vi "VI Main 1.1GPIB.vi"() -> ()   [LabVIEW 2014]
uses:
  <vilib>/Utility/file.llb/Write To Spreadsheet File (DBL).vi
  <vilib>/Analysis/NI_AALPro.lvlib
panel:
  in  "Save to File":bool
  in  "file path (dialog if empty)":path
  in  "clear graph at start":bool=TRUE
  in  "clear graph":bool
  out "Elapsed Time":dbl=5.100291728973389 format="%<%H:%M:%S>t"
  out "Measuring!":bool
  out "Current Interval":i32=2
  out "Benchmark (s)":dbl=1.077 format="%.2g"
  out "Start time":timestamp=timestamp(3634319869.0891385 s since 1904-01-01)
  in  "STOP acq":bool
  in  "# of Intervals":i32=20 min=2 step=1
  in  "Interval (s)":dbl=3.0 min=1.0 step=1.0
  in  "Quick Acq":bool
  in  "Multi Acq":bool
  in  "Reset":bool
  in  "Single Acq":bool
  in  "stop":bool
  out "intercept":dbl=5.632151768673284e-07 format="%_4g"
  out "Waveform Chart":dbl(graph)=1498.8953969009954
  out "Res. (ohm)":dbl=1498.8953969009954 format="%#.5g"
  out "XY Graph":cluster{dbl[], "Best Linear Fit":dbl[]}[](graph)=[{[0.0, 0.05050000175833702, 0.10100000351667404, 0.15150000154972076, 0.20200000703334808, 0.2524999976158142, 0.30300000309944153, 0.35350000858306885, 0.40400001406669617, 0.4544999897480011, 0.5049999952316284, 0.5554999709129333, 0.6060000061988831, 0.656499981880188, 0.7070000171661377, 0.7574999928474426, 0.8080000281333923, 0.8585000038146973, 0.9089999794960022, 0.9595000147819519, 1.0099999904632568, 1.0605000257492065, 1.1109999418258667, 1.1614999771118164, 1.2120000123977661, 1.2625000476837158, 1.312999963760376, 1.3634999990463257, 1.4140000343322754, 1.4644999504089355, 1.5149999856948853, 1.565500020980835, 1.6160000562667847, 1.6664999723434448, 1.7170000076293945, 1.7675000429153442, 1.8179999589920044, 1.868499994277954, 1.9190000295639038, 1.969499945640564, 2.0199999809265137, 2.070499897003174, 2.121000051498413, 2.1714999675750732, 2.2219998836517334, 2.2725000381469727, 2.322999954223633, 2.373500108718872, 2.4240000247955322, 2.4744999408721924, 2.5255000591278076, 2.5759999752044678, 2.626499891281128, 2.677000045776367, 2.7274999618530273, 2.7780001163482666, 2.8285000324249268, 2.878999948501587, 2.929500102996826, 2.9800000190734863, 3.0304999351501465, 3.0810000896453857, 3.131500005722046, 3.181999921798706, 3.2325000762939453, 3.2829999923706055, 3.3334999084472656, 3.384000062942505, 3.434499979019165, 3.484999895095825, 3.5355000495910645, 3.5859999656677246, 3.6364998817443848, 3.687000036239624, 3.737499952316284, 3.7880001068115234, 3.8385000228881836, 3.8889999389648438, 3.939500093460083, 3.990000009536743, 4.040500164031982, 4.091000080108643, 4.141499996185303, 4.191999912261963, 4.242499828338623, 4.293000221252441, 4.343500137329102, 4.394000053405762, 4.444499969482422, 4.494999885559082, 4.545499801635742, 4.5960001945495605, 4.646500110626221, 4.697000026702881, 4.747499942779541, 4.797999858856201, 4.848499774932861, 4.89900016784668, 4.94950008392334, 5.0], "Best Linear Fit"=[2.9321361694201187e-07, 3.4316144592594355e-05, 6.788442260585725e-05, 0.00010163152910536155, 0.0001353666593786329, 0.0001692490477580577, 0.00020289691747166216, 0.0002365230757277459, 0.0002702110796235502, 0.0003039317671209574, 0.0003375497763045132, 0.00037135041202418506, 0.00040501810144633055, 0.000438651826698333, 0.0004723611054942012, 0.0005059913382865489, 0.0005397166823968291, 0.0005734616424888372, 0.0006071235402487218, 0.0006408520275726914, 0.000674474285915494, 0.0007079437491483986, 0.0007418016903102398, 0.0007753406534902751, 0.0008092316566035151, 0.0008428616565652192, 0.0008766247192397714, 0.0009101884788833559, 0.0009441068395972252, 0.000977773917838931, 0.0010113242315128446, 0.00104525254573673, 0.0010786742204800248, 0.0011119291884824634, 0.0011458882363513112, 0.0011792887235060334, 0.0012128128437325358, 0.001246674102731049, 0.0012809749459847808, 0.0013138956855982542, 0.0013484194641932845, 0.0013821402098983526, 0.001415521022863686, 0.0014488088199868798, 0.0014823464443907142, 0.0015171199338510633, 0.0015507071511819959, 0.0015843959990888834, 0.0016174258198589087, 0.001652282546274364, 0.001685628667473793, 0.001718429964967072, 0.0017526380252093077, 0.0017857326893135905, 0.0018194534350186586, 0.001854273141361773, 0.0018880483694374561, 0.0019207267323508859, 0.0019549881108105183, 0.001989204902201891, 0.0020224947948008776, 0.002056337194517255, 0.0020900650415569544, 0.0021233297884464264, 0.0021574627608060837, 0.0021917179692536592, 0.0022237151861190796, 0.002258580643683672, 0.0022912463173270226, 0.0023252873215824366, 0.0023596647661179304, 0.0023923530243337154, 0.0024269770365208387, 0.0024603772908449173, 0.002494191052392125, 0.0025280059780925512, 0.0025607654824852943, 0.0025952423457056284, 0.0026286595966666937, 0.0026625576429069042, 0.002696041017770767, 0.002730145351961255, 0.0027635691221803427, 0.0027978394646197557, 0.00283193145878613, 0.0028640953823924065, 0.002898684237152338, 0.0029313690029084682, 0.002965638181194663, 0.0029995907098054886, 0.0030326275154948235, 0.0030669174157083035, 0.003100987756624818, 0.003135110717266798, 0.0031680287793278694, 0.0032008818816393614, 0.0032355813309550285, 0.003269442357122898, 0.0033022440038621426, 0.0033363213296979666]}, {[0.0, 0.05050000175833702, 0.10100000351667404, 0.15150000154972076, 0.20200000703334808, 0.2524999976158142, 0.30300000309944153, 0.35350000858306885, 0.40400001406669617, 0.4544999897480011, 0.5049999952316284, 0.5554999709129333, 0.6060000061988831, 0.656499981880188, 0.7070000171661377, 0.7574999928474426, 0.8080000281333923, 0.8585000038146973, 0.9089999794960022, 0.9595000147819519, 1.0099999904632568, 1.0605000257492065, 1.1109999418258667, 1.1614999771118164, 1.2120000123977661, 1.2625000476837158, 1.312999963760376, 1.3634999990463257, 1.4140000343322754, 1.4644999504089355, 1.5149999856948853, 1.565500020980835, 1.6160000562667847, 1.6664999723434448, 1.7170000076293945, 1.7675000429153442, 1.8179999589920044, 1.868499994277954, 1.9190000295639038, 1.969499945640564, 2.0199999809265137, 2.070499897003174, 2.121000051498413, 2.1714999675750732, 2.2219998836517334, 2.2725000381469727, 2.322999954223633, 2.373500108718872, 2.4240000247955322, 2.4744999408721924, 2.5255000591278076, 2.5759999752044678, 2.626499891281128, 2.677000045776367, 2.7274999618530273, 2.7780001163482666, 2.8285000324249268, 2.878999948501587, 2.929500102996826, 2.9800000190734863, 3.0304999351501465, 3.0810000896453857, 3.131500005722046, 3.181999921798706, 3.2325000762939453, 3.2829999923706055, 3.3334999084472656, 3.384000062942505, 3.434499979019165, 3.484999895095825, 3.5355000495910645, 3.5859999656677246, 3.6364998817443848, 3.687000036239624, 3.737499952316284, 3.7880001068115234, 3.8385000228881836, 3.8889999389648438, 3.939500093460083, 3.990000009536743, 4.040500164031982, 4.091000080108643, 4.141499996185303, 4.191999912261963, 4.242499828338623, 4.293000221252441, 4.343500137329102, 4.394000053405762, 4.444499969482422, 4.494999885559082, 4.545499801635742, 4.5960001945495605, 4.646500110626221, 4.697000026702881, 4.747499942779541, 4.797999858856201, 4.848499774932861, 4.89900016784668, 4.94950008392334, 5.0], "Best Linear Fit"=[5.632151768673284e-07, 3.425469348999516e-05, 6.794617180312299e-05, 0.00010163764763089373, 0.00013532912842937865, 0.0001690205992864352, 0.00020271208008492013, 0.00023640356088340506, 0.00027009504168188996, 0.0003037865025975182, 0.0003374779833960031, 0.00037116944431163135, 0.0004048609449929729, 0.00043855240590860115, 0.0004722439065899428, 0.000505935367505571, 0.0005396268681869126, 0.0005733183291025409, 0.0006070097900181691, 0.0006407012906995107, 0.0006743927516151388, 0.0007080842522964805, 0.0007417756734463953, 0.0007754671741277369, 0.0008091586748090786, 0.0008428501754904202, 0.000876541596640335, 0.0009102330973216766, 0.0009439245980030183, 0.000977616019152933, 0.0010113075198342747, 0.0010449990205156163, 0.001078690521196958, 0.0011123819423468728, 0.0011460734430282144, 0.001179764943709556, 0.0012134563648594707, 0.0012471478655408123, 0.001280839366222154, 0.0013145307873720688, 0.0013482222880534104, 0.0013819137092033252, 0.0014156052894160936, 0.0014492967105660085, 0.0014829881317159233, 0.0015166797119286917, 0.0015503711330786066, 0.001584062713291375, 0.0016177541344412898, 0.0016514455555912046, 0.0016854706906080038, 0.0017191621117579187, 0.0017528535329078335, 0.001786545113120602, 0.0018202365342705167, 0.0018539281144832852, 0.0018876195356332, 0.0019213109567831148, 0.001955002536995883, 0.001988693958145798, 0.0020223853792957127, 0.0020560769595084813, 0.002089768380658396, 0.002123459801808311, 0.002157151382021079, 0.0021908428031709943, 0.002224534224320909, 0.0022582258045336775, 0.002291917225683592, 0.002325608646833507, 0.0023593002270462754, 0.00239299164819619, 0.002426683069346105, 0.0024603746495588733, 0.0024940660707087883, 0.0025277576509215565, 0.0025614490720714716, 0.002595140493221386, 0.002628832073434155, 0.0026625234945840694, 0.002696215074796838, 0.0027299064959467527, 0.0027635979170966677, 0.0027972893382465823, 0.0028309807593964974, 0.002864672498672119, 0.0028983639198220342, 0.002932055340971949, 0.002965746762121864, 0.0029994381832717785, 0.0030331296044216935, 0.0030668213436973154, 0.0031005127648472304, 0.003134204185997145, 0.0031678956071470596, 0.0032015870282969747, 0.0032352784494468893, 0.0032689701887225115, 0.003302661609872426, 0.003336353031022341]}]
  in  "Sense range":i32(slide)
  in  "Stop (V)":dbl=5.0 format="%.4f"
  in  "Source compliance (A)":dbl=0.01 format="%.4f"
  in  "Direction":i32(slide)
  in  "Ranging":i32(slide)
  in  "Start (V)":dbl step=1.0 format="%.4p"
  in  "# of points to acquire":i32=50 min=1 max=2500 step=1
  in  "Speed":i32(slide)=2
  out "status":i32 format="%.0x"
  in  "resource name 2":string="GPIB0::24::INSTR"
  out "Qrun":bool
  out "Mrun":bool
  out "Srun":bool
  # ">"
  # "by L.Andrzejewski\nlandrzej@uottawa.ca"
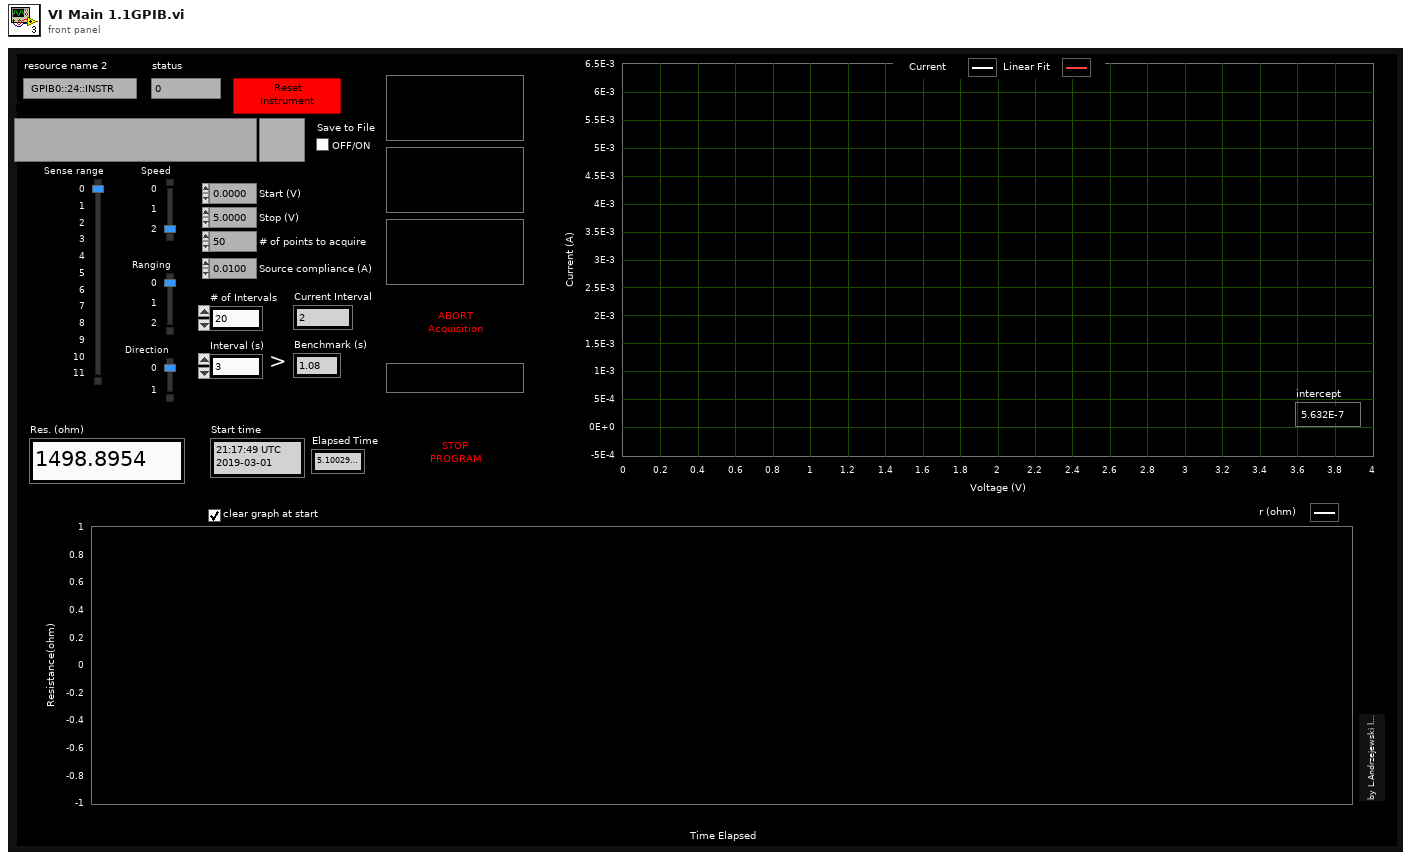
[diagram p1: front panel]
types:
  T1 = enum8{"Enabled", "Disabled", "Disabled and Grayed Out"}
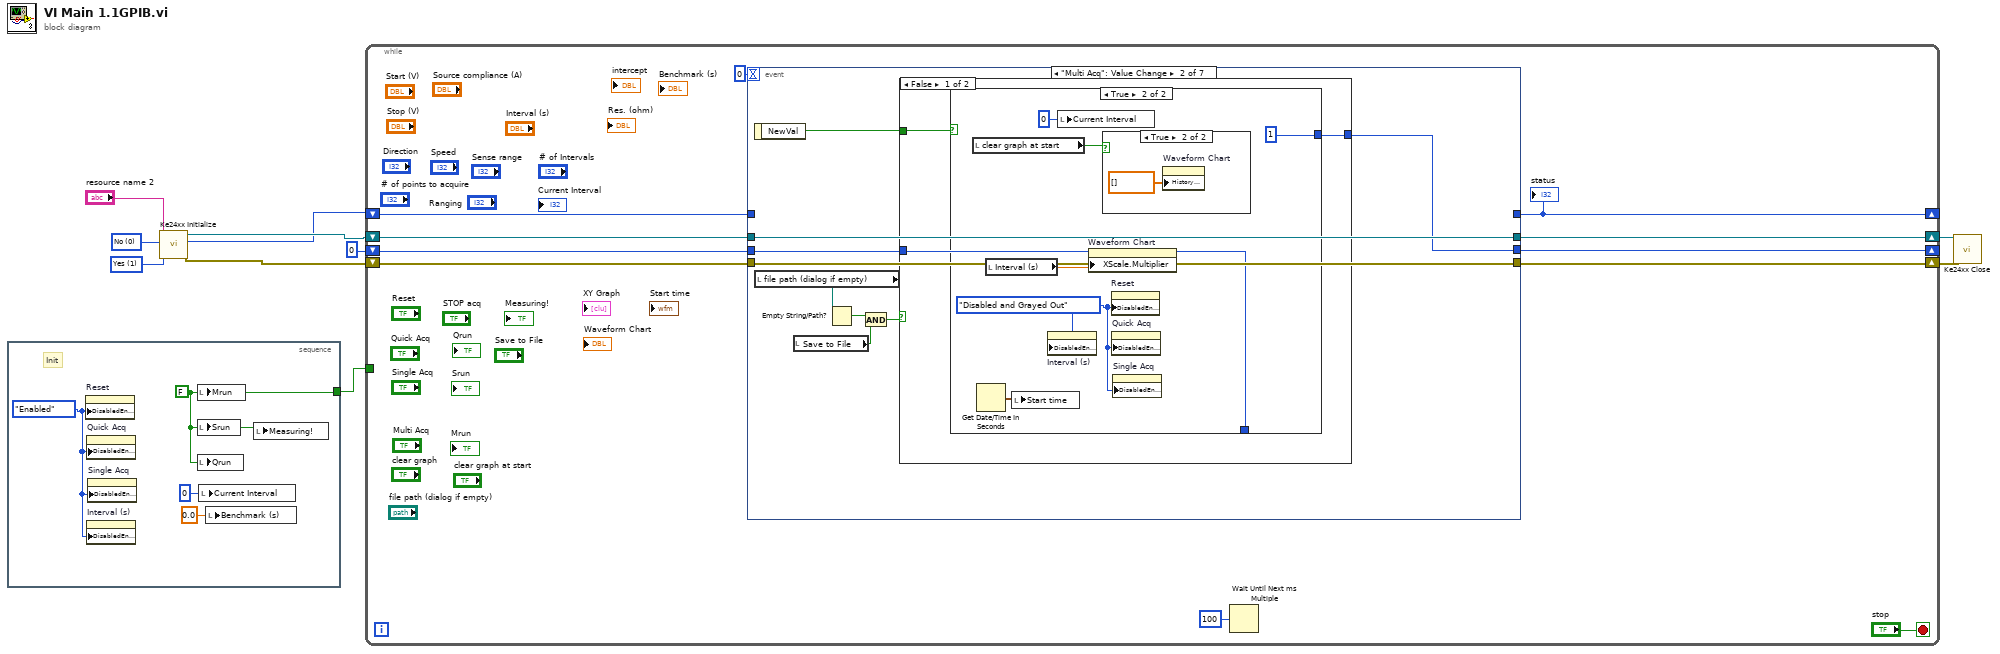
[diagram p0: block diagram]
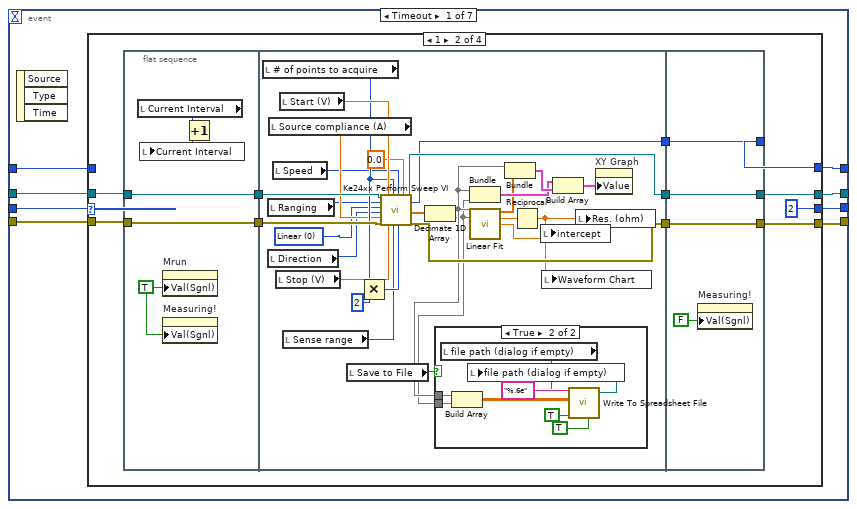
[diagram p2: hidden frame]
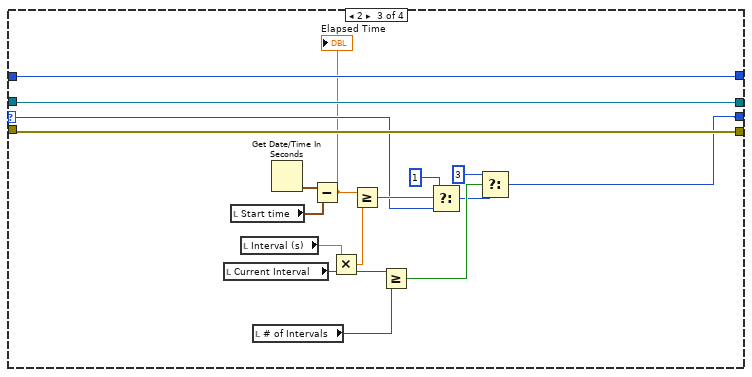
[diagram p5: hidden frame]
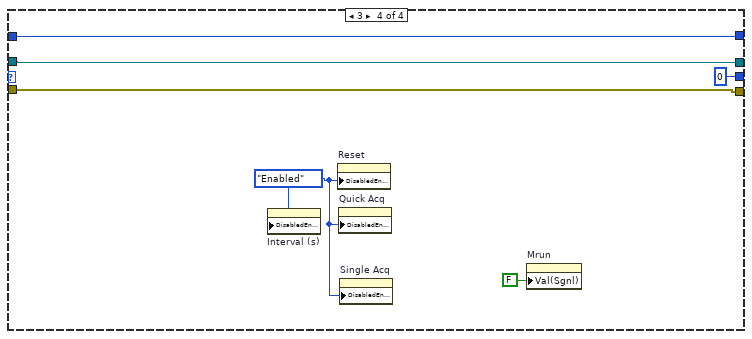
[diagram p6: hidden frame]
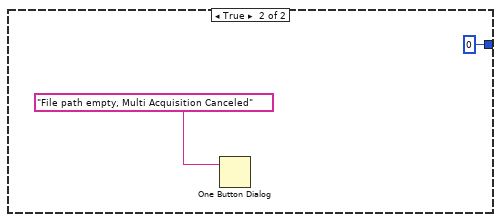
[diagram p9: hidden frame]
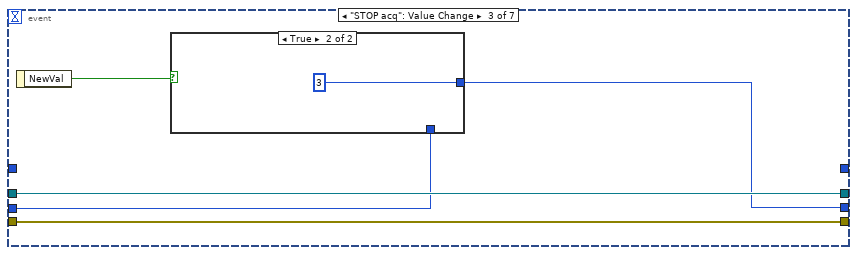
[diagram p10: hidden frame]
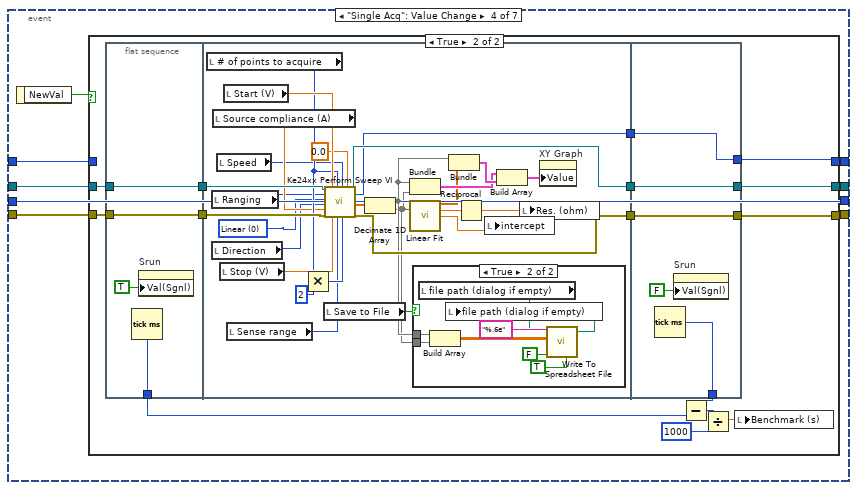
[diagram p12: hidden frame]
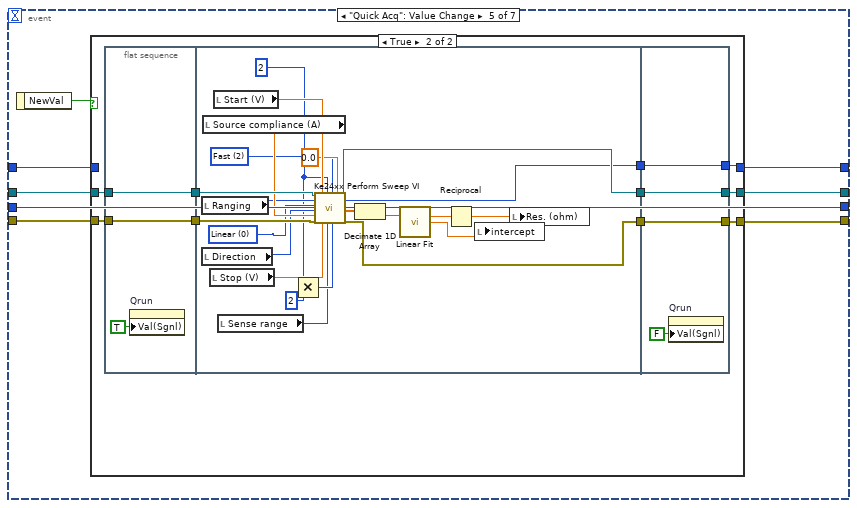
[diagram p15: hidden frame]
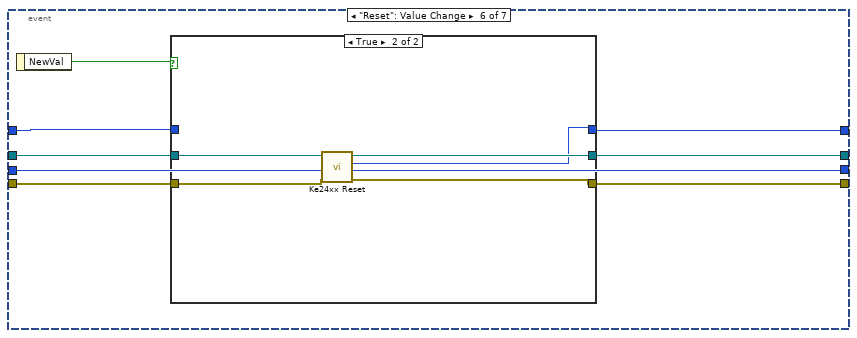
[diagram p17: hidden frame]
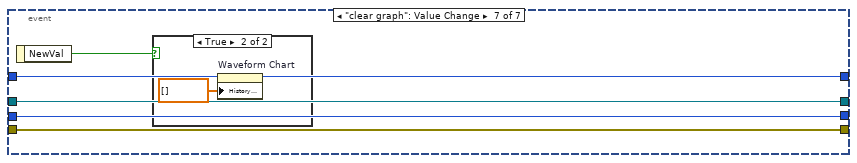
[diagram p19: hidden frame]
diagram:
  w9 = u16 1 items=["Yes"=1, "No"=0] ("id query")
  w10 = u16 0 items=["Yes"=1, "No"=0] ("reset device")
  n1 = stacked-sequence {
    tunnel: [w12] -> w3
    frame #0 {
      w11 = T1."Enabled" ("Disabled")
      w12 = FALSE ("Mrun")
      # "Init"
      n2 = property on="Reset" class="Bool"("DisabledEnum"=w11) -> ()  [unwired: 2 in, 2 out]
      n3 = property on="Quick Acq" class="Bool"("DisabledEnum"=w11) -> ()  [unwired: 2 in, 2 out]
      n4 = property on="Interval (s)" class="DigNum (strict)"("DisabledEnum"=w11) -> ()  [unwired: 2 in, 2 out]
      n5 = property on="Single Acq" class="Bool"("DisabledEnum"=w11) -> ()  [unwired: 2 in, 2 out]
      n6 = local write "Mrun"(w12) -> ()
      n7 = local write "Srun"(w12) -> ()
      n8 = local write "Qrun"(w12) -> ()
      n9 = local write "Current Interval"(0 ("Current Interval")) -> ()
      n10 = local write "Benchmark (s)"(0.0 ("Benchmark (s)")) -> ()
      n11 = local write "Measuring!"(w12) -> ()
    }
  }
  n12 = call "Ke24xx Initialize.vi"("reset device"=w10, "id query"=w9, "resource name"="resource name 2") -> ("error out"=w4:errorcluster, "status"=w5:i32, "instrument handle out"=w6:refnum<visa-resource-name>)  [unwired: 6 in]
  n13 = while {
    shift-right: [w20] -> w8
    shift-left: w6 -> [w22]
    shift-right: [w19] -> w7
    shift-left: w4 -> [w21]
    shift-right: [w17] -> _
    shift-left: w5 -> [w18]
    tunnel: w3 -> [_]
    shift-right: [w15] -> _
    shift-left: 0 -> [w16]
    stop <- "stop" stop-if-true
    n14 = event shown="[1] \"Multi Acq\": Value Change" {
      selector: _ -> [_ _ _ _ _ _ _]
      dyn-events: _ -> [_ _ _ _ _ _ _]
      timeout: 0 -> [_ _ _ _ _ _ _]
      tunnel: [w29 w124 w142 w149 w220 w271 w286] -> w20
      tunnel: w22 -> [w32 w124 w142 w152 w223 w272 w286]
      tunnel: [w28 w123 w141 w150 w221 w270 w284] -> w19
      tunnel: w21 -> [w31 w123 w141 w151 w222 w269 w284]
      tunnel: w18 -> [w30 _ _ w148 w219 w274 w287]
      tunnel: [w26 _ _ w147 w218 w273 w287] -> w17
      tunnel: w16 -> [w33 w121 w139 w146 w217 w268 w285]
      tunnel: [w27 w122 w140 w146 w217 w268 w285] -> w15
      event Timeout {
        n15 = event-data() -> ()  [unwired: 1 in, 3 out]
        n16 = case shown="1" w33 {
          selector: w33 -> [w34 _ w99 _]
          tunnel: w32 -> [w36 w46 w108 w114]
          tunnel: w31 -> [w35 w45 w109 w112]
          tunnel: w30 -> [w37 _ w110 w115]
          tunnel: [w36 w44 w108 w114] -> w29
          tunnel: [w35 w43 w109 w112] -> w28
          tunnel: [w34 2 w96 0 ("t")] -> w27
          tunnel: [w37 w41 w110 w115] -> w26
          frame 0, Default {
          }
          frame 1 {
            n17 = flat-sequence {
              tunnel: w45 -> [w52]
              tunnel: w46 -> [w53]
              tunnel: [w53] -> w48
              tunnel: [w52] -> w47
              tunnel: w48 -> [w76]
              tunnel: w47 -> [w75]
              tunnel: [w74] -> w40
              tunnel: [w73] -> w39
              tunnel: [w58] -> w38
              tunnel: [w91] -> w41
              tunnel: [w92] -> w44
              tunnel: [w93] -> w43
              tunnel: w40 -> [w93]
              tunnel: w39 -> [w92]
              tunnel: w38 -> [w91]
              frame #0 {
                w49 = TRUE ("Value (Signaling)")
                n18 = local read "Current Interval"() -> (w50:i32)
                n19 = property on="Mrun" class="Bool (strict)"("Val(Sgnl)"=w49) -> ()  [unwired: 2 in, 2 out]
                n20 = property on="Measuring!" class="Bool (strict)"("Val(Sgnl)"=w49) -> ()  [unwired: 2 in, 2 out]
                n21 = Increment(x=w50) -> (x+1=w51:i32)
                n22 = local write "Current Interval"(w51) -> ()
              }
              frame #1 {
                w60 = 0 items=["Linear", "Logarithmic"] ("spacing")
                n23 = local read "# of points to acquire"() -> (w67:i32)
                n24 = local read "Ranging"() -> (w62:i32)
                n25 = local read "Direction"() -> (w61:i32)
                n26 = local read "Source compliance (A)"() -> (w64:dbl)
                n27 = local read "Speed"() -> (w63:i32)
                n28 = local read "Stop (V)"() -> (w69:dbl)
                n29 = local read "Start (V)"() -> (w70:dbl)
                n30 = local read "Sense range"() -> (w65:i32)
                n31 = local read "Save to File"() -> (w56:bool)
                n32 = Multiply(x=w67, y=2) -> (x*y=w66:i32)
                n33 = call "Ke24xx Perform Sweep VI.vi"("instrument handle"=w76, "ranging"=w62, "spacing"=w60, "direction"=w61, "source compliance"=w64, "error in (no error)"=w75, "start"=w70, "stop"=w69, "number of points"=w67, "sense range"=w65, "speed"=w63, "size of reading"=w66, "source protection"=0.0) -> ("instrument handle out"=w73:refnum<visa-resource-name>, "status"=w58:i32, "out"=w77:dbl[], "error out"=w74:errorcluster)  [unwired: 3 in]
                n34 = Decimate 1D Array(w77) -> (w55:dbl[], w54:dbl[])
                n35 = case shown="True" w56 {
                  tunnel: w55 -> [_ w89]
                  tunnel: w54 -> [_ w88]
                  frame False {
                  }
                  frame True {
                    n36 = local read "file path (dialog if empty)"() -> (w85:path)
                    n37 = Build Array(w89, w88) -> (w84:dbl[][])
                    n38 = call-poly <vilib>:"Write To Spreadsheet File.vi"("transpose? (no:F)"=TRUE, "format (%.3f)"="%.6e", "append to file? (new file:F)"=TRUE, "2D data"=w84, "file path (dialog if empty)"=w85) -> ("new file path (Not A Path if cancelled)"=w83:path)  [unwired: 3 in]
                    n39 = local write "file path (dialog if empty)"(w83) -> ()
                  }
                }
                n40 = Bundle(w55, w54) -> (w80:cluster{dbl[], dbl[]})  [unwired: 1 in]
                n41 = call <vilib>:"Linear Fit.vi"("Y"=w54, "X"=w55) -> ("Best Linear Fit"=w79:dbl[], "slope"=w78:dbl, "intercept"=w72:dbl)  [unwired: 9 in, 2 out]
                n42 = Bundle(w55, "Best Linear Fit"=w79) -> (w81:cluster{dbl[], "Best Linear Fit":dbl[]})  [unwired: 1 in]
                n43 = Reciprocal(x=w78) -> (1/x=w57:dbl)
                n44 = local write "intercept"(w72) -> ()
                n45 = local write "Waveform Chart"(w57) -> ()
                n46 = Build Array(w80, w81) -> (w71:cluster{dbl[], "Best Linear Fit":dbl[]}[])
                n47 = local write "Res. (ohm)"(w57) -> ()
                n48 = property on="XY Graph" class="XYGraph (strict)"("Value"=w71) -> ()  [unwired: 2 in, 2 out]
              }
              frame #2 {
                n49 = property on="Measuring!" class="Bool (strict)"("Val(Sgnl)"=FALSE ("Value (Signaling)")) -> ()  [unwired: 2 in, 2 out]
              }
            }
          }
          frame 2 {
            n50 = local read "Current Interval"() -> (w102:i32)
            n51 = local read "Start time"() -> (w106:timestamp)
            n52 = local read "Interval (s)"() -> (w105:dbl)
            n53 = local read "# of Intervals"() -> (w101:i32)
            n54 = Get Date/Time In Seconds() -> (seconds since 1Jan1904=w107:timestamp)
            n55 = Subtract(x=w107, y=w106) -> (x-y=w94:dbl)
            "Elapsed Time" <- w94
            n56 = Multiply(x=w105, y=w102) -> (x*y=w104:dbl)
            n57 = Greater Or Equal?(x=w94, y=w104) -> (x >= y?=w103:bool)
            n58 = Greater Or Equal?(x=w102, y=w101) -> (x >= y?=w98:bool)
            n59 = Select(t=1, s=w103, f=w99) -> (s? t:f=w97:i32)
            n60 = Select(t=3, s=w98, f=w97) -> (s? t:f=w96:i32)
          }
          frame 3 {
            w111 = T1."Enabled" ("Disabled")
            n61 = property on="Interval (s)" class="DigNum (strict)"("DisabledEnum"=w111) -> ()  [unwired: 2 in, 2 out]
            n62 = property on="Reset" class="Bool"("DisabledEnum"=w111) -> ()  [unwired: 2 in, 2 out]
            n63 = property on="Quick Acq" class="Bool"("DisabledEnum"=w111) -> ()  [unwired: 2 in, 2 out]
            n64 = property on="Single Acq" class="Bool"("DisabledEnum"=w111) -> ()  [unwired: 2 in, 2 out]
            n65 = property on="Mrun" class="Bool (strict)"("Val(Sgnl)"=FALSE ("Value (Signaling)")) -> ()  [unwired: 2 in, 2 out]
          }
        }
      }
      event "Multi Acq": Value Change {
        n66 = event-data() -> ("NewVal"=w125:bool)  [unwired: 1 in]
        n67 = local read "file path (dialog if empty)"() -> (w120:path)
        n68 = local read "Save to File"() -> (w117:bool)
        n69 = Empty String/Path?(string/path=w120) -> (empty?=w119:bool)
        n70 = And(x=w119, y=w117) -> (x .and. y?=w118:bool)
        n71 = case shown="False" w118 {
          tunnel: w125 -> [w128 _]
          tunnel: [w127 0] -> w122
          tunnel: w121 -> [w126 _]
          frame False {
            n72 = case shown="True" w128 {
              tunnel: [w129 1] -> w127
              tunnel: w126 -> [w129 _]
              frame False {
              }
              frame True {
                w132 = T1."Disabled and Grayed Out" ("Disabled")
                n73 = local read "clear graph at start"() -> (w131:bool)
                n74 = Get Date/Time In Seconds() -> (seconds since 1Jan1904=w134:timestamp)
                n75 = local read "Interval (s)"() -> (w133:dbl)
                n76 = local write "Start time"(w134) -> ()
                n77 = property on="Interval (s)" class="DigNum (strict)"("DisabledEnum"=w132) -> ()  [unwired: 2 in, 2 out]
                n78 = local write "Current Interval"(0 ("Current Interval")) -> ()
                n79 = property on="Waveform Chart" class="WFChart (strict)"("XScale.Multiplier"=w133) -> ()  [unwired: 2 in, 2 out]
                n80 = case shown="True" w131 {
                  frame False {
                  }
                  frame True {
                    n81 = property on="Waveform Chart" class="WFChart (strict)"("History Data"=dbl[] []) -> ()  [unwired: 2 in, 2 out]
                  }
                }
                n82 = property on="Reset" class="Bool"("DisabledEnum"=w132) -> ()  [unwired: 2 in, 2 out]
                n83 = property on="Quick Acq" class="Bool"("DisabledEnum"=w132) -> ()  [unwired: 2 in, 2 out]
                n84 = property on="Single Acq" class="Bool"("DisabledEnum"=w132) -> ()  [unwired: 2 in, 2 out]
              }
            }
          }
          frame True {
            n85 = One Button Dialog(message="File path empty, Multi Acquisition Canceled") -> ()  [unwired: 1 in, 1 out]
          }
        }
      }
      event "STOP acq": Value Change {
        n86 = event-data() -> ("NewVal"=w143:bool)  [unwired: 1 in]
        n87 = case shown="True" w143 {
          tunnel: [w144 3] -> w140
          tunnel: w139 -> [w144 _]
          frame False {
          }
          frame True {
          }
        }
      }
      event "Single Acq": Value Change {
        n88 = event-data() -> ("NewVal"=w153:bool)  [unwired: 1 in]
        n89 = case shown="True" w153 {
          tunnel: w152 -> [w156 w171]
          tunnel: w151 -> [w155 w170]
          tunnel: [w155 w169] -> w150
          tunnel: [w156 w168] -> w149
          tunnel: [w154 w163] -> w147
          tunnel: w148 -> [w154 _]
          frame False {
          }
          frame True {
            n90 = flat-sequence {
              tunnel: w170 -> [w174]
              tunnel: w171 -> [w175]
              tunnel: [w175] -> w165
              tunnel: [w174] -> w164
              tunnel: [w172] -> w160
              tunnel: [w196] -> w167
              tunnel: [w195] -> w166
              tunnel: w165 -> [w198]
              tunnel: w164 -> [w197]
              tunnel: [w179] -> w162
              tunnel: [w215] -> w168
              tunnel: [w216] -> w169
              tunnel: w167 -> [w216]
              tunnel: w166 -> [w215]
              tunnel: [w214] -> w163
              tunnel: w162 -> [w214]
              tunnel: [w212] -> w161
              frame #0 {
                n91 = Tick Count (ms)() -> (millisecond timer value=w172:u32)
                n92 = property on="Srun" class="Bool (strict)"("Val(Sgnl)"=TRUE ("Value (Signaling)")) -> ()  [unwired: 2 in, 2 out]
              }
              frame #1 {
                w181 = 0 items=["Linear", "Logarithmic"] ("spacing")
                n93 = local read "# of points to acquire"() -> (w188:i32)
                n94 = local read "Ranging"() -> (w183:i32)
                n95 = local read "Direction"() -> (w182:i32)
                n96 = local read "Source compliance (A)"() -> (w185:dbl)
                n97 = local read "Speed"() -> (w184:i32)
                n98 = local read "Stop (V)"() -> (w190:dbl)
                n99 = local read "Start (V)"() -> (w191:dbl)
                n100 = local read "Sense range"() -> (w186:i32)
                n101 = Multiply(x=w188, y=2) -> (x*y=w187:i32)
                n102 = local read "Save to File"() -> (w176:bool)
                n103 = call "Ke24xx Perform Sweep VI.vi"("instrument handle"=w198, "ranging"=w183, "spacing"=w181, "direction"=w182, "source compliance"=w185, "error in (no error)"=w197, "start"=w191, "stop"=w190, "number of points"=w188, "sense range"=w186, "speed"=w184, "size of reading"=w187, "source protection"=0.0) -> ("instrument handle out"=w195:refnum<visa-resource-name>, "status"=w179:i32, "out"=w199:dbl[], "error out"=w196:errorcluster)  [unwired: 3 in]
                n104 = Decimate 1D Array(w199) -> (w178:dbl[], w177:dbl[])
                n105 = Bundle(w178, w177) -> (w202:cluster{dbl[], dbl[]})  [unwired: 1 in]
                n106 = call <vilib>:"Linear Fit.vi"("Y"=w177, "X"=w178) -> ("Best Linear Fit"=w201:dbl[], "slope"=w200:dbl, "intercept"=w194:dbl)  [unwired: 9 in, 2 out]
                n107 = case shown="True" w176 {
                  tunnel: w178 -> [_ w211]
                  tunnel: w177 -> [_ w210]
                  frame False {
                  }
                  frame True {
                    n108 = local read "file path (dialog if empty)"() -> (w207:path)
                    n109 = Build Array(w211, w210) -> (w206:dbl[][])
                    n110 = call-poly <vilib>:"Write To Spreadsheet File.vi"("transpose? (no:F)"=TRUE, "format (%.3f)"="%.6e", "append to file? (new file:F)"=FALSE, "2D data"=w206, "file path (dialog if empty)"=w207) -> ("new file path (Not A Path if cancelled)"=w205:path)  [unwired: 3 in]
                    n111 = local write "file path (dialog if empty)"(w205) -> ()
                  }
                }
                n112 = Bundle(w178, "Best Linear Fit"=w201) -> (w203:cluster{dbl[], "Best Linear Fit":dbl[]})  [unwired: 1 in]
                n113 = Reciprocal(x=w200) -> (1/x=w193:dbl)
                n114 = local write "intercept"(w194) -> ()
                n115 = Build Array(w202, w203) -> (w192:cluster{dbl[], "Best Linear Fit":dbl[]}[])
                n116 = local write "Res. (ohm)"(w193) -> ()
                n117 = property on="XY Graph" class="XYGraph (strict)"("Value"=w192) -> ()  [unwired: 2 in, 2 out]
              }
              frame #2 {
                n118 = Tick Count (ms)() -> (millisecond timer value=w212:u32)
                n119 = property on="Srun" class="Bool (strict)"("Val(Sgnl)"=FALSE ("Value (Signaling)")) -> ()  [unwired: 2 in, 2 out]
              }
            }
            n120 = Subtract(x=w161, y=w160) -> (x-y=w159:u32)
            n121 = Divide(x=w159, y=u32 1000) -> (x/y=w157:dbl)
            n122 = local write "Benchmark (s)"(w157) -> ()
          }
        }
      }
      event "Quick Acq": Value Change {
        n123 = event-data() -> ("NewVal"=w224:bool)  [unwired: 1 in]
        n124 = case shown="True" w224 {
          tunnel: w223 -> [w227 w237]
          tunnel: w222 -> [w226 w236]
          tunnel: [w226 w235] -> w221
          tunnel: [w227 w234] -> w220
          tunnel: [w225 w229] -> w218
          tunnel: w219 -> [w225 _]
          frame False {
          }
          frame True {
            n125 = flat-sequence {
              tunnel: w236 -> [w239]
              tunnel: w237 -> [w240]
              tunnel: [w240] -> w233
              tunnel: [w239] -> w232
              tunnel: w233 -> [w259]
              tunnel: w232 -> [w258]
              tunnel: [w257] -> w231
              tunnel: [w256] -> w230
              tunnel: [w241] -> w228
              tunnel: [w266] -> w234
              tunnel: [w267] -> w235
              tunnel: w231 -> [w267]
              tunnel: w230 -> [w266]
              tunnel: [w264] -> w229
              tunnel: w228 -> [w264]
              frame #0 {
                n126 = property on="Qrun" class="Bool (strict)"("Val(Sgnl)"=TRUE ("Qrun")) -> ()  [unwired: 2 in, 2 out]
              }
              frame #1 {
                w242 = 2 items=["Slow", "Medium", "Fast"] ("speed")
                w243 = 2 ("x")
                w245 = 0 items=["Linear", "Logarithmic"] ("spacing")
                n127 = local read "Ranging"() -> (w247:i32)
                n128 = local read "Direction"() -> (w246:i32)
                n129 = local read "Source compliance (A)"() -> (w248:dbl)
                n130 = local read "Stop (V)"() -> (w252:dbl)
                n131 = local read "Start (V)"() -> (w253:dbl)
                n132 = local read "Sense range"() -> (w249:i32)
                n133 = Multiply(x=w243, y=2) -> (x*y=w250:i32)
                n134 = call "Ke24xx Perform Sweep VI.vi"("instrument handle"=w259, "ranging"=w247, "spacing"=w245, "direction"=w246, "source compliance"=w248, "error in (no error)"=w258, "start"=w253, "stop"=w252, "number of points"=w243, "sense range"=w249, "speed"=w242, "size of reading"=w250, "source protection"=0.0) -> ("instrument handle out"=w256:refnum<visa-resource-name>, "status"=w241:i32, "out"=w260:dbl[], "error out"=w257:errorcluster)  [unwired: 3 in]
                n135 = Decimate 1D Array(w260) -> (w263:dbl[], w261:dbl[])
                n136 = call <vilib>:"Linear Fit.vi"("Y"=w261, "X"=w263) -> ("slope"=w262:dbl, "intercept"=w255:dbl)  [unwired: 9 in, 3 out]
                n137 = Reciprocal(x=w262) -> (1/x=w254:dbl)
                n138 = local write "intercept"(w255) -> ()
                n139 = local write "Res. (ohm)"(w254) -> ()
              }
              frame #2 {
                n140 = property on="Qrun" class="Bool (strict)"("Val(Sgnl)"=FALSE ("Qrun")) -> ()  [unwired: 2 in, 2 out]
              }
            }
          }
        }
      }
      event "Reset": Value Change {
        n141 = event-data() -> ("NewVal"=w275:bool)  [unwired: 1 in]
        n142 = case shown="True" w275 {
          tunnel: [w278 w279] -> w273
          tunnel: w274 -> [w278 _]
          tunnel: w272 -> [w277 w283]
          tunnel: [w277 w282] -> w271
          tunnel: [w276 w280] -> w270
          tunnel: w269 -> [w276 w281]
          frame False {
          }
          frame True {
            n143 = call "Ke24xx Reset.vi"("error in (no error)"=w281, "instrument handle"=w283) -> ("error out"=w280:errorcluster, "status"=w279:i32, "instrument handle out"=w282:refnum<visa-resource-name>)  [unwired: 7 in]
          }
        }
      }
      event "clear graph": Value Change {
        n144 = event-data() -> ("NewVal"=w288:bool)  [unwired: 1 in]
        n145 = case shown="True" w288 {
          frame False {
          }
          frame True {
            n146 = property on="Waveform Chart" class="WFChart (strict)"("History Data"=dbl[] []) -> ()  [unwired: 2 in, 2 out]
          }
        }
      }
    }
    "status" <- w17
    n147 = Wait Until Next ms Multiple(millisecond multiple=u32 100) -> ()  [unwired: 1 out]
  }
  n148 = call "Ke24xx Close.vi"("error in (no error)"=w7, "instrument handle"=w8) -> ()  [unwired: 8 in, 2 out]
